vi "Helper - Modify Chart.vi"(8 "error in (no error)":errorcluster, 9 "Y Scale.Range:Maximum":dbl format="%#.6g", 10 "Y Scale.Range:Minimum":dbl format="%#.6g", 11 "Chart Reference":refnum<vi>) -> (0 "error out":errorcluster)   [LabVIEW 2019]
doc: "This VI is used as a subVI for Control References.vi. It shows how to use a control reference to change the settings of a waveform chart."
panel:
  # "Right-click a control reference and choose Select VI Server Class to specify the class of a reference type. Alternatively, you can Ctrl-Drag an existing control or indicator into a reference control to set its class type."
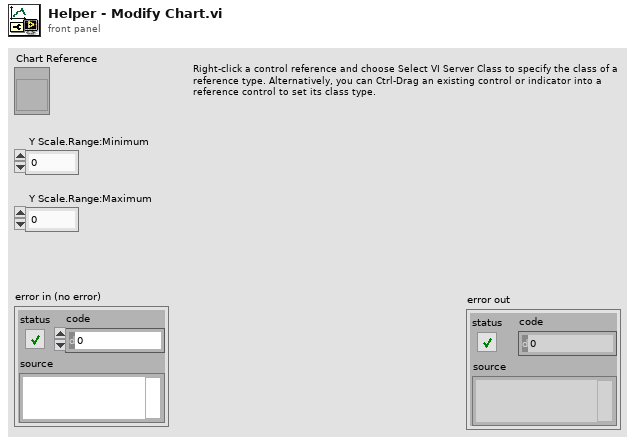
[diagram p1: front panel]
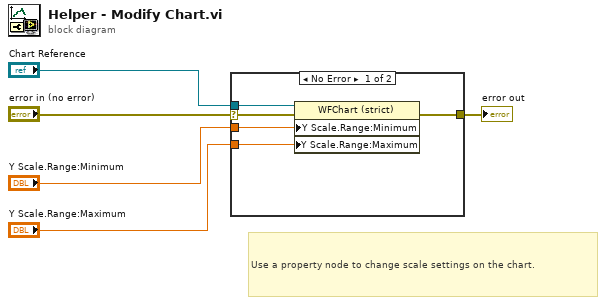
[diagram p0: block diagram]
diagram:
  # "Use a property node to change scale settings on the chart."
  n1 = case shown="No Error" "error in (no error)" {
    selector: "error in (no error)" -> [w8 w11]
    tunnel: "Y Scale.Range:Maximum" -> [w6 _]
    tunnel: "Y Scale.Range:Minimum" -> [w7 _]
    tunnel: "Chart Reference" -> [w10 _]
    tunnel: [w9 w11] -> w2
    frame No Error {
      n2 = property class="WFChart (strict)"(reference=w10, error in=w8, "Y Scale.Range:Minimum"=w7, "Y Scale.Range:Maximum"=w6) -> (error out=w9:errorcluster)  [unwired: 1 out]
    }
    frame Error {
    }
  }
  "error out" <- w2
